vi "UT_004_LV to TOML.vi"() -> ()   [LabVIEW 2020]
uses:
  <vilib>/addons/_JKI Toolkits/Caraya/classes/Assert/Assert True.vi
  <vilib>/addons/_JKI Toolkits/Caraya/classes/Test/Test.lvclass
  lib/TOML.lvlib
  <vilib>/addons/_JKI Toolkits/Caraya/classes/Assert/Assert.lvclass
panel:
  out "toml String 3":string
  out "toml String 2":string
  out "toml String":string
  out "error out 3":errorcluster
  out "error out":errorcluster
  out "error out 2":errorcluster
  in  "data 3":string[][](array[string])=[["a", "b"], ["d", "e"], ["g", "h"]]
  in  "data 2":string[][](array[string])=[["a", "b", "c"], ["d", "e", "f"]]
  in  "data":string[][](array[string])=[["a", "b", "c"], ["d", "e", "f"], ["g", "h", "i"]]
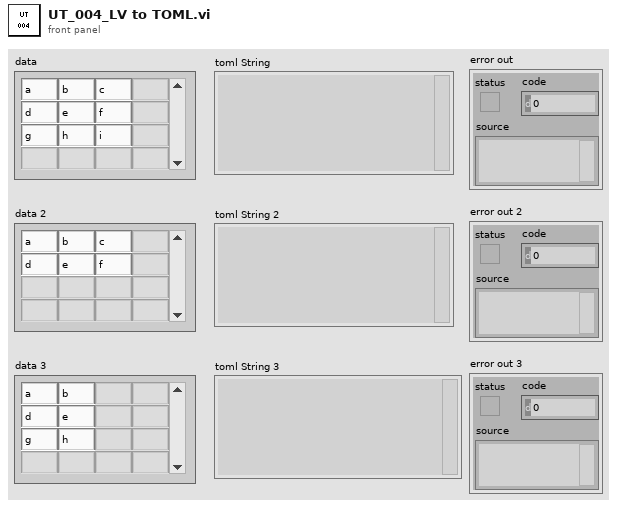
[diagram p1: front panel]
types:
  T1 = typedef "TOML.lvlib/TOML Value.ctl" = cluster{"type":enum16{"Table", "Array", "String", "Integer", "Float", "Boolean", "Offset Date-Time", "Local Date-Time", "Local Date", "Local Time", "Path"}, "value":variant}
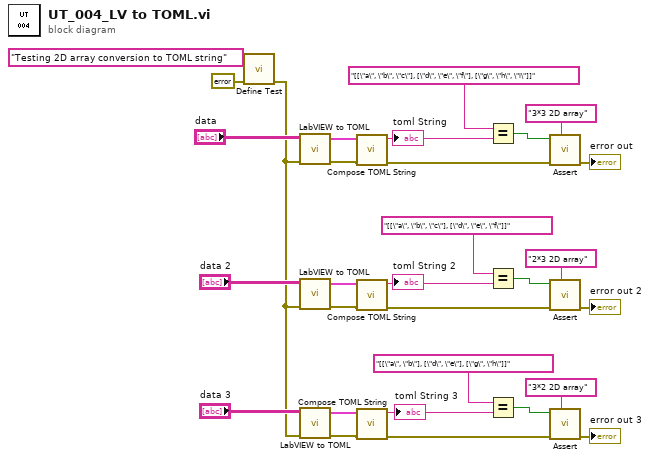
[diagram p0: block diagram]
diagram:
  n1 = call <vilib>:"Define Test.vi"("error in (no error)"=errorcluster {"status"=FALSE, "code"=0, "source"=""}, "Label (VI Title)"="Testing 2D array conversion to TOML string") -> ("error out"=w13:errorcluster)  [unwired: 8 in, 1 out]
  n2 = call "LabVIEW to TOML.vi"("error in (no error)"=w13, "LV Value"="data") -> ("error out"=w1:errorcluster, "TOML Value"=w2:T1)  [unwired: 7 in, 1 out]
  n3 = call "LabVIEW to TOML.vi"("error in (no error)"=w13, "LV Value"="data 2") -> ("error out"=w4:errorcluster, "TOML Value"=w3:T1)  [unwired: 7 in, 1 out]
  n4 = call "LabVIEW to TOML.vi"("error in (no error)"=w13, "LV Value"="data 3") -> ("error out"=w15:errorcluster, "TOML Value"=w16:T1)  [unwired: 7 in, 1 out]
  n5 = call "Compose TOML String.vi"("error in (no error)"=w1, "Value"=w2) -> ("error out"=w22:errorcluster, "String"=w23:string)  [unwired: 8 in]
  "toml String" <- w23
  n6 = call "Compose TOML String.vi"("error in (no error)"=w4, "Value"=w3) -> ("error out"=w26:errorcluster, "String"=w7:string)  [unwired: 8 in]
  "toml String 2" <- w7
  n7 = call "Compose TOML String.vi"("error in (no error)"=w15, "Value"=w16) -> ("error out"=w18:errorcluster, "String"=w6:string)  [unwired: 8 in]
  "toml String 3" <- w6
  n8 = Equal?(x="[[\"a\", \"b\", \"c\"], [\"d\", \"e\", \"f\"], [\"g\", \"h\", \"i\"]]", y=w23) -> (x = y?=w5:bool)
  n9 = Equal?(x="[[\"a\", \"b\", \"c\"], [\"d\", \"e\", \"f\"]]", y=w7) -> (x = y?=w25:bool)
  n10 = Equal?(x="[[\"a\", \"b\"], [\"d\", \"e\"], [\"g\", \"h\"]]", y=w6) -> (x = y?=w19:bool)
  n11 = call-poly <vilib>:"Assert.vi"("Label"="3*3 2D array" ("Label (VI Title)"), "error in (no error)"=w22, "True?"=w5) -> ("error out"=→"error out":errorcluster)  [unwired: 7 in, 1 out]
  n12 = call-poly <vilib>:"Assert.vi"("Label"="2*3 2D array" ("Label (VI Title)"), "error in (no error)"=w26, "True?"=w25) -> ("error out"=→"error out 2":errorcluster)  [unwired: 7 in, 1 out]
  n13 = call-poly <vilib>:"Assert.vi"("Label"="3*2 2D array" ("Label (VI Title)"), "error in (no error)"=w18, "True?"=w19) -> ("error out"=→"error out 3":errorcluster)  [unwired: 7 in, 1 out]
